vi "Lock-In Analysis.vi"(0 "Signal in":dbl[][](array[numeric])=array6x5000[30000 elements], 1 "Phase&Tc In":T1(array[cluster])=[{"Phase"=0.0, "Time constant"=0.1, "Set Tc"=FALSE, "Autophase"=FALSE, "Order"=2.0}, {"Phase"=0.0, "Time constant"=0.1, "Set Tc"=FALSE, "Autophase"=FALSE, "Order"=2.0}, {"Phase"=0.0, "Time constant"=0.1, "Set Tc"=FALSE, "Autophase"=FALSE, "Order"=2.0}, {"Phase"=0.0, "Time constant"=0.1, "Set Tc"=FALSE, "Autophase"=FALSE, "Order"=2.0}, {"Phase"=0.0, "Time constant"=0.1, "Set Tc"=FALSE, "Autophase"=FALSE, "Order"=2.0}, {"Phase"=0.0, "Time constant"=0.1, "Set Tc"=FALSE, "Autophase"=FALSE, "Order"=2.0}, {"Phase"=0.0, "Time constant"=0.1, "Set Tc"=FALSE, "Autophase"=FALSE, "Order"=2.0}, {"Phase"=0.0, "Time constant"=0.1, "Set Tc"=FALSE, "Autophase"=FALSE, "Order"=2.0}, {"Phase"=0.0, "Time constant"=0.1, "Set Tc"=FALSE, "Autophase"=FALSE, "Order"=2.0}, {"Phase"=0.0, "Time constant"=0.1, "Set Tc"=FALSE, "Autophase"=FALSE, "Order"=2.0}, {"Phase"=0.0, "Time constant"=0.1, "Set Tc"=FALSE, "Autophase"=FALSE, "Order"=2.0}, {"Phase"=0.0, "Time constant"=0.1, "Set Tc"=FALSE, "Autophase"=FALSE, "Order"=2.0}, {"Phase"=0.0, "Time constant"=0.1, "Set Tc"=FALSE, "Autophase"=FALSE, "Order"=2.0}, {"Phase"=0.0, "Time constant"=0.1, "Set Tc"=FALSE, "Autophase"=FALSE, "Order"=2.0}, {"Phase"=0.0, "Time constant"=0.1, "Set Tc"=FALSE, "Autophase"=FALSE, "Order"=2.0}, {"Phase"=0.0, "Time constant"=0.1, "Set Tc"=FALSE, "Autophase"=FALSE, "Order"=2.0}, {"Phase"=0.0, "Time constant"=0.1, "Set Tc"=FALSE, "Autophase"=FALSE, "Order"=2.0}] {"Phase" min=0.0 max=360.0 scale=0.0..360.0}, 5 "AI Block Size In":i32=5000, 7 "Results":dbl[][](array[numeric])=[[1.1085752698169061e-06, 8.970523484593692e-07, 1.426058219262487e-06, 38.9795731407906], [0.009851325382064164, -0.0009794262328395094, 0.009899893308964286, -5.677731707079707], [1.3085970697368273e-06, 7.35860824175527e-07, 1.5013052466038e-06, 29.35026849878307], [2.653910755996262e-06, 1.0145343098285082e-06, 2.8412184299366806e-06, 20.9208047375633], [-6.086289413703597e-07, 1.180787094252328e-06, 1.3284153530528245e-06, 117.2685442231227], [2.777937660299593e-06, 8.877049230863689e-07, 2.9163260577278655e-06, 17.721560078700946]], 9 "AI Rate In":dbl=10000.0 format="%.2f", 11 "OSC Configuration In":T2(array[cluster])=[[{"Signal Type"=enum."Sine Wave", "DC"=0.0, "Amplitude"=0.001, "frequency"=2.0, "Phase"=0.0}, {"Signal Type"=enum."Sine Wave", "DC"=0.0, "Amplitude"=0.0, "frequency"=2.0, "Phase"=0.0}, {"Signal Type"=enum."Sine Wave", "DC"=0.0, "Amplitude"=0.0, "frequency"=20.0, "Phase"=0.0}], [{"Signal Type"=enum."Sine Wave", "DC"=0.0, "Amplitude"=0.0, "frequency"=2.0, "Phase"=0.0}, {"Signal Type"=enum."Sine Wave", "DC"=0.0, "Amplitude"=0.0, "frequency"=2.0, "Phase"=0.0}, {"Signal Type"=enum."Sine Wave", "DC"=0.0, "Amplitude"=0.0, "frequency"=20.0, "Phase"=0.0}]] {"frequency" step=0.001 format="%.3p"; "Amplitude" format="%0.2p"; "DC" min=-0.99 max=0.99 format="%.2p"}, 12 "Phase Log In":dbl[](array[numeric])=[0.9999999999893834, 0.9999999999893834]) -> (4 "Demodulation Out":dbl[][](array[numeric])=[[0.032308985716257205, -0.0020089800684537727, 0.032371384878394444, -3.5583001590229886], [0.023385861272623584, -0.0014539178662531169, 0.02343101330770514, -3.5574201885889787], [-3.111140914765216e-05, 2.7289487058700542e-06, 3.123206852318323e-05, -5.0131650508604935], [-3.1370210865590166e-05, 3.1631661467659442e-06, 3.1532606636697875e-05, -5.751181571584788]], 6 "Phase Log Out":dbl[](array[numeric]), 8 "Phase&Tc Out":T1(array[cluster]))   [LabVIEW 2011, in "Lock-In Variable Channels_2.lvclass"]
uses:
  Lock-In Variable Channels_2.lvclass
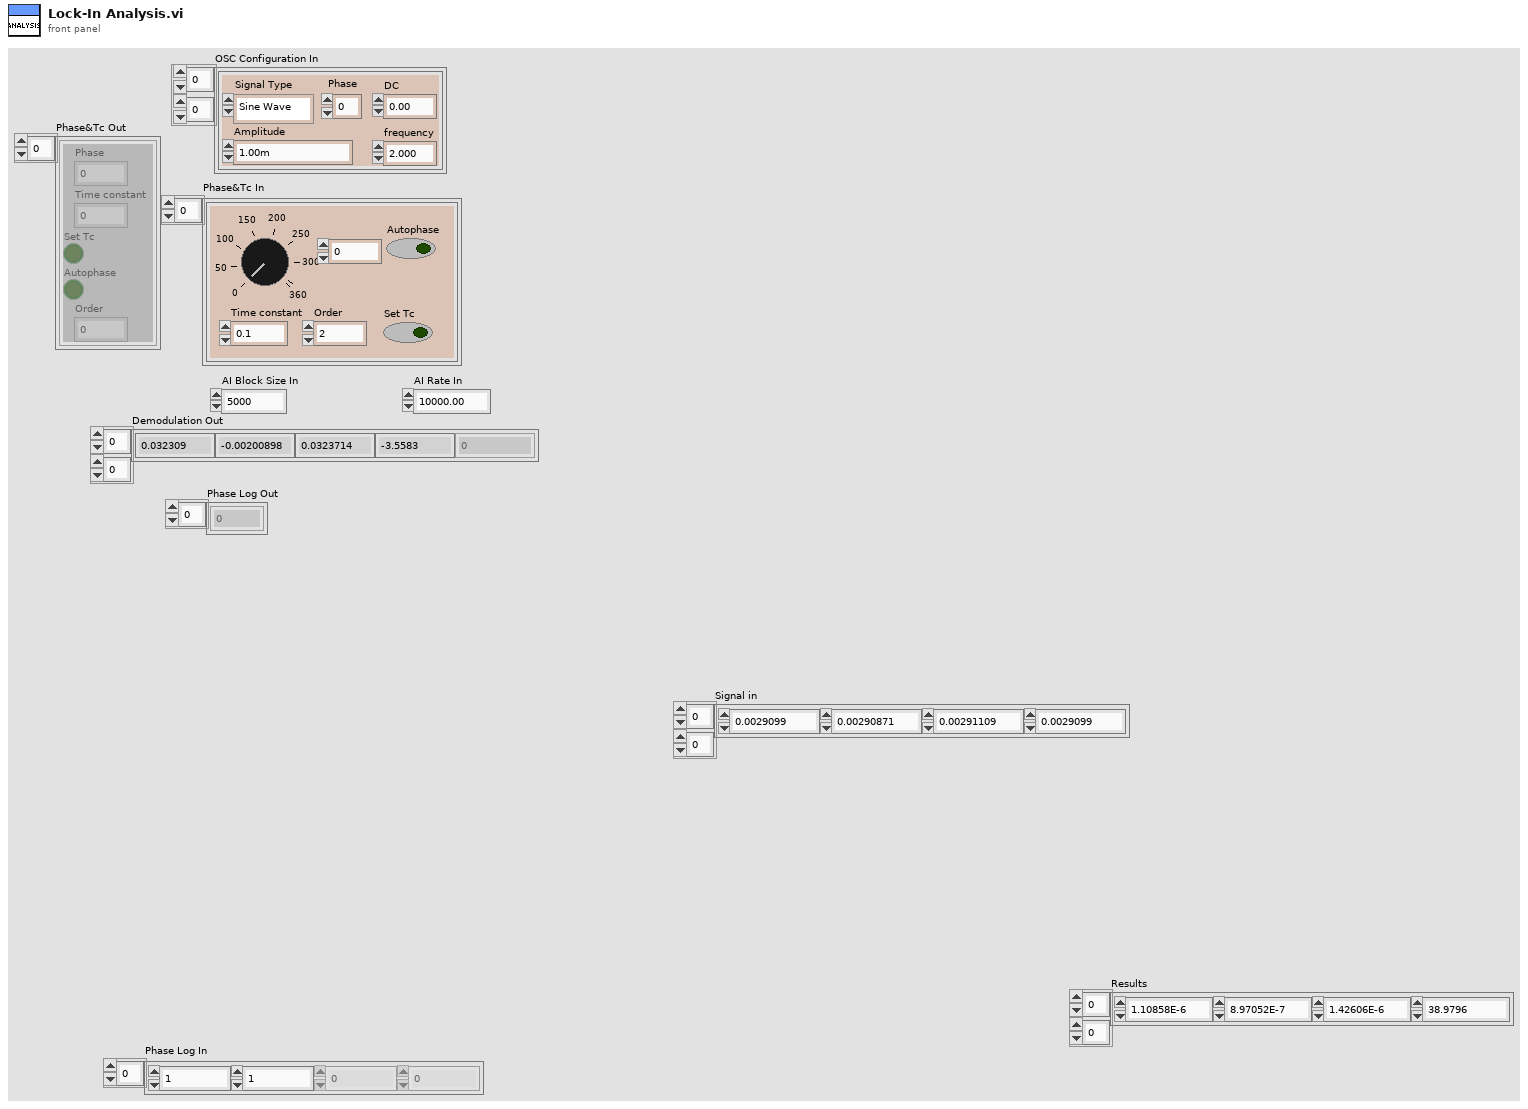
[diagram p1: front panel]
types:
  T1 = cluster{"Phase":dbl, "Time constant":dbl, "Set Tc":bool, "Autophase":bool, "Order":dbl}[]
  T2 = cluster{"Signal Type":enum16{"Sine Wave", "Triangle Wave", "Square Wave", "Sawtooth Wave"}, "DC":dbl, "Amplitude":dbl, "frequency":dbl, "Phase":dbl}[][]
  T3 = cluster{"Ref X":dbl[], "Ref Y":dbl[], "AI Rate":dbl, "AI Block Size":dbl, "Frequency":dbl, "Ref amp":dbl}[]
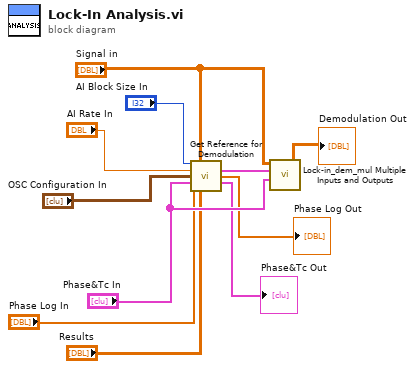
[diagram p0: block diagram]
diagram:
  n1 = call "Get Reference for Demodulation.vi"("AI Block Size"="AI Block Size In", "Signal"="Signal in", "AI Rate"="AI Rate In", "OSC Configuration"="OSC Configuration In", "Phase&Tc"="Phase&Tc In", "phase log"="Phase Log In", "Results"="Results") -> ("Ref In"=w7:T3, "Phase Log Out"=→"Phase Log Out":dbl[], "Phase&Tc Out"=→"Phase&Tc Out":T1)  [unwired: 6 in]
  n2 = call "Lock-in_dem_mul Multiple Inputs and Outputs.vi"("Phase&Tc"="Phase&Tc In", "Ref in"=w7, "Signal"="Signal in") -> ("Demodulation"=→"Demodulation Out":dbl[][])  [unwired: 2 in]
